vi "BinaryFormatSaveLoop.vi"(7 "Controls ref.":T2, 8 "data error in":errorcluster, 9 "data queue in":refnum<queue>, 11 "control queue in":refnum<queue>) -> (0 "queue error out":errorcluster, 1 "error out":errorcluster, 2 "Quit Binary":bool, 3 "Format":T1=enum."Binary Files")   [LabVIEW 2014]
uses:
  WriterState.ctl
  <instrlib>/GenericDAQ/VI/GenericDAQ_Signal.ctl
  SaveControlsRef.ctl
  ControlDef/Files_Format.ctl
  BinaryHeader.ctl
  <instrlib>/GenericDAQ/GenericDAQ.lvlib
panel:
  out "Numeric":i32
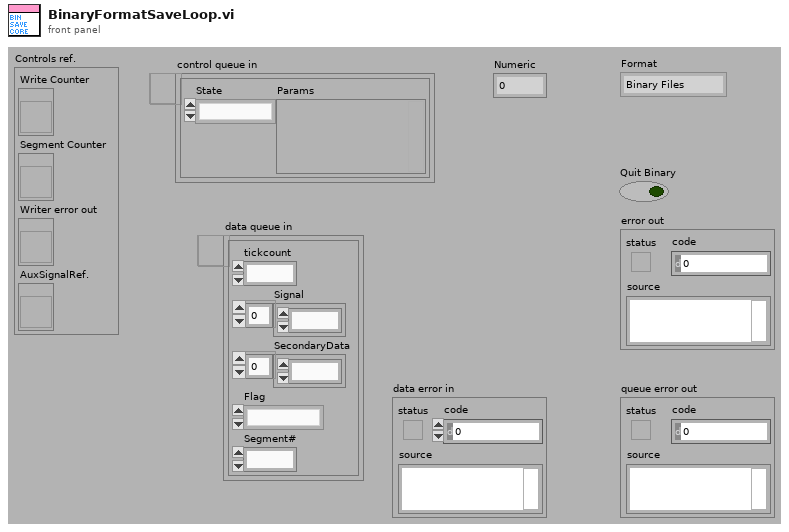
[diagram p1: front panel]
types:
  T1 = typedef "Files_Format.ctl" = enum16{"Text Files", "mzML Files", "Binary Files", "BioMap Files", "imzML Files"}
  T2 = typedef "SaveControlsRef.ctl" = cluster{"Write Counter":refnum<vi>, "Segment Counter":refnum<vi>, "Writer error out":refnum<vi>, "AuxSignalRef.":refnum<vi>}
  T3 = enum16{"open", "replace", "create", "open or create", "replace or create", "replace or create with confirmation"}
  T4 = enum16{"big-endian, network order", "native, host order", "little-endian"}
  T5 = typedef "BinaryHeader.ctl" = cluster{"Start Position":dbl[], "StepWidth":dbl[], "Dimension":i32[], "SpecLength":i32}
  T6 = typedef "WriterState.ctl" = cluster{"State":enum16{"Open", "Close", "ChangeFormat", "SetHeader", "QuitProg."}, "Params":variant}
  T7 = enum16{"Open", "Close", "ChangeFormat", "SetHeader", "QuitProg."}
  T8 = typedef "GenericDAQ.lvlib/GenericDAQ_Signal.ctl" = cluster{"tickcount":u32, "Signal":sgl[], "SecondaryData":dbl[], "Flag":enum16{"Normal", "LineStart", "LineEnd", "FrameStart", "FrameEnd", "Reserved1", "Reserved2"}, "Segment#":i32}
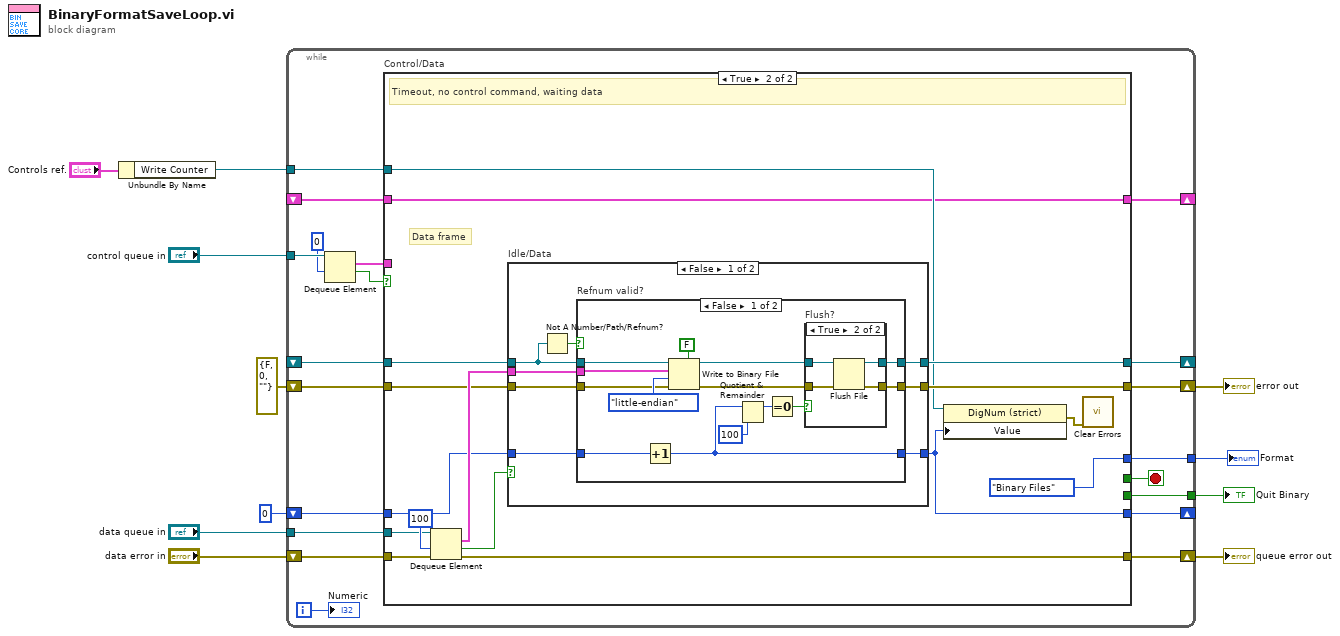
[diagram p0: block diagram]
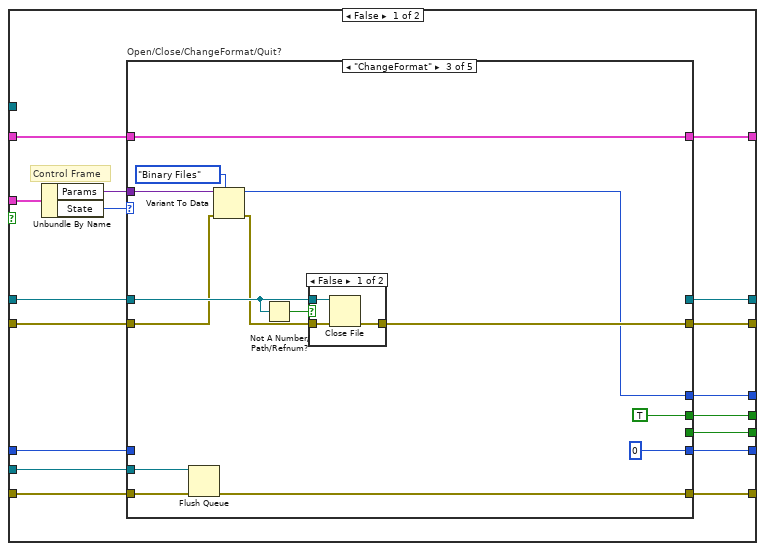
[diagram p2: hidden frame]
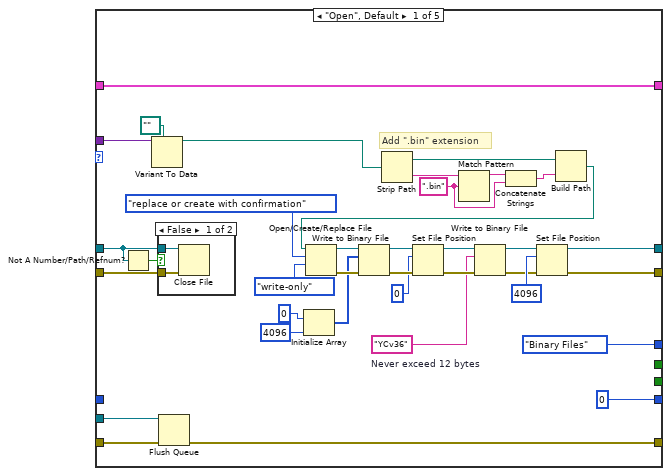
[diagram p3: hidden frame]
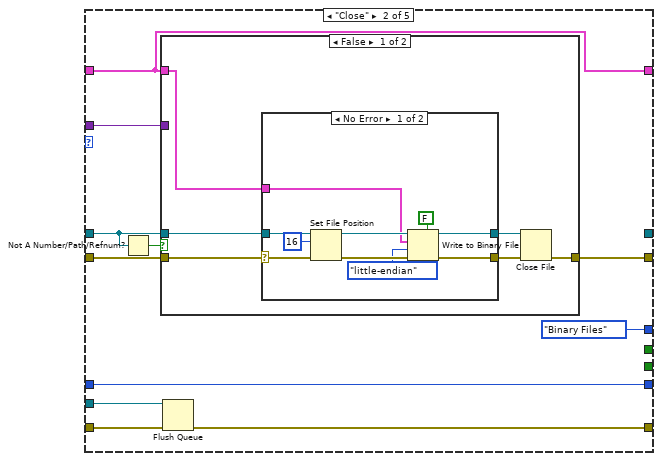
[diagram p5: hidden frame]
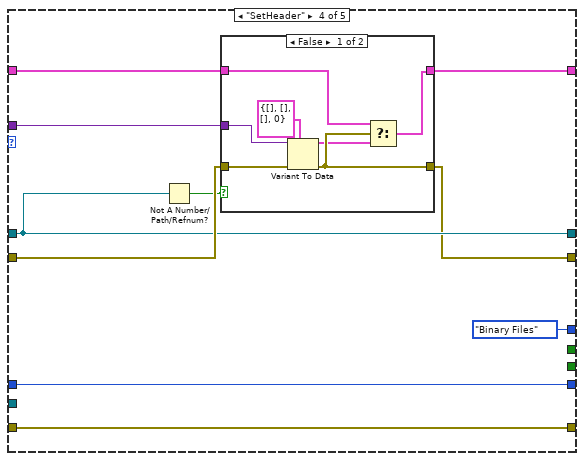
[diagram p9: hidden frame]
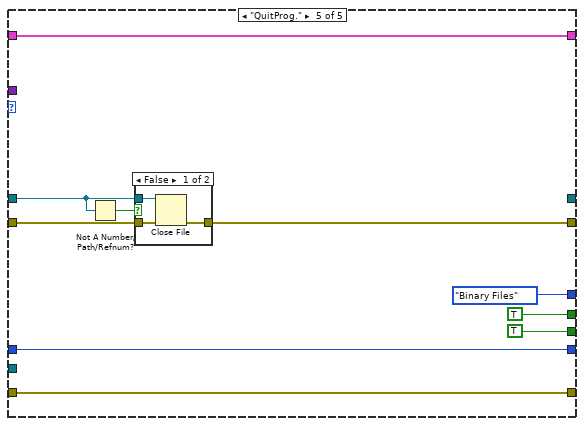
[diagram p11: hidden frame]
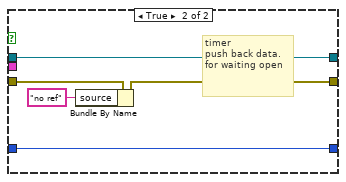
[diagram p14: hidden frame]
diagram:
  n1 = Unbundle By Name("Controls ref.") -> ("Write Counter"=w2:refnum<vi>)
  n2 = while {
    tunnel: [w25] -> w6
    shift-right: [w26] -> _
    shift-left: 0 -> [w31]
    tunnel: "data queue in" -> [w21]
    shift-right: [w29] -> _
    shift-left: _ -> [w30]
    tunnel: "control queue in" -> [w24]
    tunnel: [w17] -> w1
    shift-right: [w28] -> w5
    shift-left: errorcluster {"status"=FALSE, "code"=0, "source"=""} ("error out") -> [w27]
    tunnel: w2 -> [w15]
    shift-right: [w16] -> w11
    shift-left: "data error in" -> [w20]
    shift-right: [w14] -> _
    shift-left: _ -> [w13]
    i -> [w12]
    stop <- w18 stop-if-true
    n3 = Dequeue Element(queue=w24, timeout in ms (-1)=0) -> (element=w19:T6, timed out?=w22:bool)  [unwired: 1 in, 2 out]
    n4 = case "Control/Data" shown="True" w22 {
      tunnel: w31 -> [w37 w175]
      tunnel: w30 -> [w44 w178]
      tunnel: [w43 w177] -> w29
      tunnel: [w42 w176] -> w28
      tunnel: w27 -> [w45 w179]
      tunnel: [w38 w171] -> w26
      tunnel: [w41 _] -> w25
      tunnel: w21 -> [w35 w182]
      tunnel: w20 -> [w36 w181]
      tunnel: w19 -> [w48 _]
      tunnel: [w40 _] -> w18
      tunnel: [w39 Files_Format."Binary Files" ("Format")] -> w17
      tunnel: [w34 w173] -> w16
      tunnel: w15 -> [_ w172]
      tunnel: [w33 w170] -> w14
      tunnel: w13 -> [w32 w170]
      frame False {
        # "Control Frame"
        n5 = Unbundle By Name(w48) -> ("Params"=w46:variant, "State"=w47:T7)
        n6 = case "Open/Close/ChangeFormat/Quit?" shown="\"ChangeFormat\"" w47 {
          tunnel: w46 -> [w61 w89 w122 w142 _]
          tunnel: w45 -> [w83 w90 w119 w143 w158]
          tunnel: w44 -> [w82 w96 w128 w141 w157]
          tunnel: [w74 _ _ w141 _] -> w43
          tunnel: [w68 w94 w126 w140 w159] -> w42
          tunnel: [_ _ _ _ TRUE] -> w41
          tunnel: [_ _ TRUE _ TRUE] -> w40
          tunnel: [Files_Format."Binary Files" ("Format") Files_Format."Binary Files" ("Format") w121 Files_Format."Binary Files" ("Format") Files_Format."Binary Files" ("Format")] -> w39
          tunnel: [0 w95 0 w144 w161] -> w38
          tunnel: w37 -> [_ w95 _ w144 w161]
          tunnel: w36 -> [w77 w93 w124 w136 w156]
          tunnel: w35 -> [w76 w91 w125 _ _]
          tunnel: [w75 w92 w123 w136 w156] -> w34
          tunnel: [w49 w88 w118 w138 w155] -> w33
          tunnel: w32 -> [w49 w88 w118 w139 w155]
          frame "Open", Default {
            w50 = "YCv36"  # Never exceed 12 bytes
            w67 = ".bin" ("regular expression")
            # "Add \".bin\" extension"
            n7 = Not A Number/Path/Refnum?(number/path/refnum=w82) -> (NaN/Path/Refnum?=w84:bool)
            n8 = Variant To Data(type=path "" ("path"), Variant=w61) -> (data=w59:path)  [unwired: 1 in, 1 out]
            n9 = case shown="False" w84 {
              tunnel: w83 -> [w86 _]
              tunnel: w82 -> [w85 _]
              frame False {
                n10 = Close File(refnum=w85, error in=w86) -> ()  [unwired: 2 out]
              }
              frame True {
              }
            }
            n11 = Flush Queue(queue=w76, error in (no error)=w77) -> (error out=w75:errorcluster)  [unwired: 2 out]
            n12 = Initialize Array(u8 0 ("offset (in bytes) (0)"), 4096 ("dimension size")) -> (w56:u8[])
            n13 = Strip Path(path=w59) -> (stripped path=w63:path, name=w64:string)
            n14 = Match Pattern(string=w64, regular expression=w67) -> (before substring=w66:string)  [unwired: 1 in, 3 out]
            n15 = Concatenate Strings(w66, w67) -> (w65:string)
            n16 = Build Path(base path=w63, name or relative path=w65) -> (appended path=w62:path)
            n17 = Open/Create/Replace File(file path (use dialog)=w62, operation (0:open)=T3."replace or create with confirmation", access (0:read/write)=enum16{"read/write", "read-only", "write-only"}."write-only") -> (refnum out=w73:refnum<file>, error out=w69:errorcluster)  [unwired: 3 in, 1 out]
            n18 = Write to Binary File(file (use dialog)=w73, data=w56, error in=w69) -> (refnum out=w52:refnum<file>, error out=w53:errorcluster)  [unwired: 3 in, 1 out]
            n19 = Set File Position(offset (in bytes) (0)=i64 0, refnum=w52, error in=w53) -> (refnum out=w55:refnum<file>, error out=w54:errorcluster)  [unwired: 1 in]
            n20 = Write to Binary File(file (use dialog)=w55, data=w50, error in=w54) -> (refnum out=w57:refnum<file>, error out=w58:errorcluster)  [unwired: 3 in, 1 out]
            n21 = Set File Position(offset (in bytes) (0)=i64 4096, refnum=w57, error in=w58) -> (refnum out=w74:refnum<file>, error out=w68:errorcluster)  [unwired: 1 in]
          }
          frame "Close" {
            n22 = Not A Number/Path/Refnum?(number/path/refnum=w96) -> (NaN/Path/Refnum?=w97:bool)
            n23 = case shown="False" w97 {
              tunnel: w90 -> [w99 w116]
              tunnel: w96 -> [w102 _]
              tunnel: [w103 w116] -> w94
              tunnel: w89 -> [_ _]
              tunnel: w88 -> [w98 _]
              frame False {
                n24 = case shown="No Error" w99 {
                  selector: w99 -> [w108 w114]
                  tunnel: w102 -> [w113 w115]
                  tunnel: [w111 w115] -> w101
                  tunnel: [w110 w114] -> w100
                  tunnel: w98 -> [w104 _]
                  frame No Error {
                    n25 = Set File Position(offset (in bytes) (0)=i64 16, refnum=w113, error in=w108) -> (refnum out=w112:refnum<file>, error out=w109:errorcluster)  [unwired: 1 in]
                    n26 = Write to Binary File(file (use dialog)=w112, data=w104, error in=w109, 5:FALSE ("prepend array or string size? (T)"), 9:T4."little-endian" ("byte order (0:big-endian, network order)")) -> (refnum out=w111:refnum<file>, error out=w110:errorcluster)  [unwired: 1 in, 1 out]
                  }
                  frame Error {
                  }
                }
                n27 = Close File(refnum=w101, error in=w100) -> (error out=w103:errorcluster)  [unwired: 1 out]
              }
              frame True {
              }
            }
            n28 = Flush Queue(queue=w91, error in (no error)=w93) -> (error out=w92:errorcluster)  [unwired: 2 out]
          }
          frame "ChangeFormat" {
            n29 = Flush Queue(queue=w125, error in (no error)=w124) -> (error out=w123:errorcluster)  [unwired: 2 out]
            n30 = Variant To Data(error in=w119, type=Files_Format."Binary Files" ("Format"), Variant=w122) -> (data=w121:T1, error out=w120:errorcluster)
            n31 = Not A Number/Path/Refnum?(number/path/refnum=w128) -> (NaN/Path/Refnum?=w129:bool)
            n32 = case shown="False" w129 {
              tunnel: w120 -> [w133 w134]
              tunnel: w128 -> [w132 _]
              tunnel: [w131 w134] -> w126
              frame False {
                n33 = Close File(refnum=w132, error in=w133) -> (error out=w131:errorcluster)  [unwired: 1 out]
              }
              frame True {
              }
            }
          }
          frame "SetHeader" {
            n34 = Not A Number/Path/Refnum?(number/path/refnum=w141) -> (NaN/Path/Refnum?=w137:bool)
            n35 = case shown="False" w137 {
              tunnel: w143 -> [w151 w152]
              tunnel: w142 -> [w150 _]
              tunnel: [w148 w152] -> w140
              tunnel: w139 -> [w146 w153]
              tunnel: [w145 w153] -> w138
              frame False {
                n36 = Variant To Data(error in=w151, type=T5 {"Start Position"=[], "StepWidth"=[], "Dimension"=[], "SpecLength"=0} ("output cluster"), Variant=w150) -> (data=w147:T5, error out=w148:errorcluster)
                n37 = Select(t=w146, s=w148, f=w147) -> (s? t:f=w145:T5)
              }
              frame True {
              }
            }
          }
          frame "QuitProg." {
            n38 = Not A Number/Path/Refnum?(number/path/refnum=w157) -> (NaN/Path/Refnum?=w160:bool)
            n39 = case shown="False" w160 {
              tunnel: w158 -> [w166 w167]
              tunnel: w157 -> [w165 _]
              tunnel: [w164 w167] -> w159
              frame False {
                n40 = Close File(refnum=w165, error in=w166) -> (error out=w164:errorcluster)  [unwired: 1 out]
              }
              frame True {
              }
            }
          }
        }
      }
      frame True {
        # "Data frame"
        # "Timeout, no control command, waiting data"
        n41 = Dequeue Element(queue=w182, timeout in ms (-1)=100, error in (no error)=w181) -> (element=w180:T8, timed out?=w174:bool, error out=w173:errorcluster)  [unwired: 1 out]
        n42 = case "Idle/Data" shown="False" w174 {
          tunnel: w180 -> [w191 _]
          tunnel: w179 -> [w190 w218]
          tunnel: w178 -> [w188 w219]
          tunnel: [w185 w219] -> w177
          tunnel: [w184 w218] -> w176
          tunnel: w175 -> [w187 w217]
          tunnel: [w186 w217] -> w171
          frame False {
            n43 = Not A Number/Path/Refnum?(number/path/refnum=w188) -> (NaN/Path/Refnum?=w189:bool)
            n44 = case "Refnum valid?" shown="False" w189 {
              tunnel: [w193 w214] -> w184
              tunnel: [w194 w216] -> w185
              tunnel: w191 -> [w203 _]
              tunnel: w188 -> [w202 w216]
              tunnel: w190 -> [w201 w215]
              tunnel: w187 -> [w200 w212]
              tunnel: [w197 w212] -> w186
              frame False {
                n45 = Increment(x=w200) -> (x+1=w197:i32)
                n46 = Write to Binary File(file (use dialog)=w202, data=w203, error in=w201, 5:FALSE ("prepend array or string size? (T)"), 9:T4."little-endian" ("byte order (0:big-endian, network order)")) -> (refnum out=w196:refnum<file>, error out=w195:errorcluster)  [unwired: 1 in, 1 out]
                n47 = Quotient & Remainder(x=w197, y=100) -> (x-y*floor(x/y)=w199:i32)  [unwired: 1 out]
                n48 = Equal To 0?(x=w199) -> (x = 0?=w198:bool)
                n49 = case "Flush?" shown="True" w198 {
                  tunnel: w196 -> [w207 w211]
                  tunnel: [w207 w210] -> w194
                  tunnel: w195 -> [w206 w209]
                  tunnel: [w206 w208] -> w193
                  frame False {
                  }
                  frame True {
                    n50 = Flush File(refnum=w211, error in=w209) -> (refnum out=w210:refnum<file>, error out=w208:errorcluster)
                  }
                }
              }
              frame True {
                # "timer\npush back data.\nfor waiting open"
                n51 = Bundle By Name(cluster=w215, "source"="no ref") -> (w214:errorcluster)
              }
            }
          }
          frame True {
          }
        }
        n52 = property class="DigNum (strict)"(reference=w172, "Value"=w171) -> (error out=w168:errorcluster)  [unwired: 1 in, 1 out]
        n53 = call <vilib>:"Clear Errors.vi"("error in (no error)"=w168) -> ()  [unwired: 5 in, 2 out]
      }
    }
    "Numeric" <- w12
  }
  "queue error out" <- w11
  "Quit Binary" <- w6
  "error out" <- w5
  "Format" <- w1
